vi "TagContainer-TestMain.vi"() -> ()   [LabVIEW 2017, in "TagDB(DEV).lvlib"]
uses:
  TagDB(DEV).lvlib
  a1ae43e1-b2e0-48b2-b5bf-09d8c6337ec0.vi
  5d4c14d8-f2b2-4cd0-9f9f-81160b0f88f4.vi
  69a5f5dc-289e-4520-a43d-4a6e53800127.vi
  f6a41f1a-46ba-40d5-b8b9-4f6d9d3cd2d0.vi
  b9594d6d-a8e1-4e69-b527-0d31d87043e6.vi
  _Support/DataAccess/_NameCacher.vi
  _Support/DataAccess/_datatypeChecker.vi
  _Support/DataAccess/TagDB Ref to DVR.vi
  <vilib>/Utility/Data Type/Get Type Information.vi
  <vilib>/Utility/error.llb/Trim Whitespace.vi
  _Support/Error/_[error50000]Invalid DB REF.vi
  _Support/Error/_[error50002]Invalid DataType.vi
  <userlib>/_OpenG.lib/comparison/comparison.llb/Variant Changed__ogtk.vi
  _Support/Change Detector/TagDB dbChanged.vi
panel:
  out "changed?":bool[](array[boolean])
  in  "Reject New Tag(F)":bool=TRUE
  out "should be datatype error":errorcluster
  out "should be no tag error":errorcluster
  out "Raw name":string
  in  "Type":cluster{"Numeric":i32, "String":string}
  in  "Stop":bool
  out "Value":cluster{"Numeric":i32, "String":string}
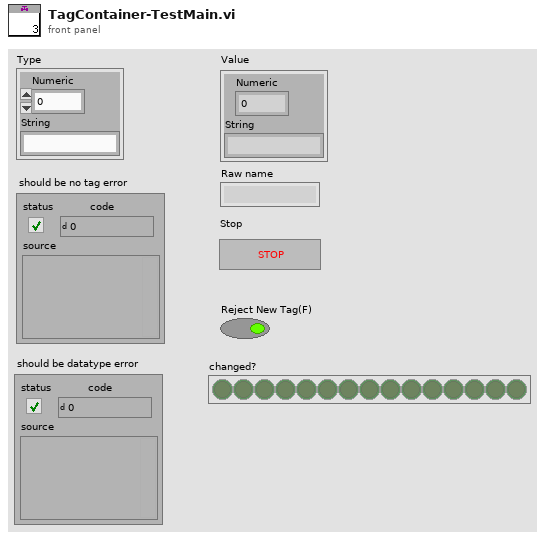
[diagram p1: front panel]
types:
  T1 = typedef "TagDB(DEV).lvlib/TagContainer.ctl" = refnum<k1>
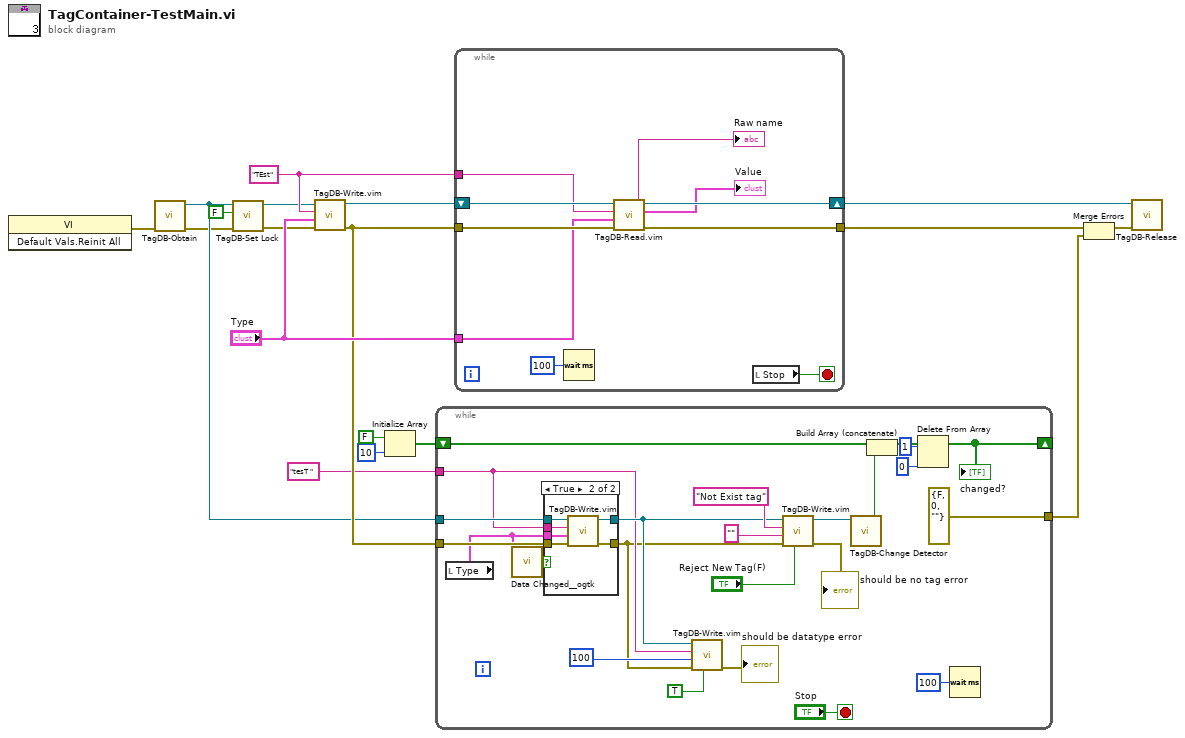
[diagram p0: block diagram]
diagram:
  w14 = "TEst" ("name")
  n1 = invoke class="VI" method="Default Vals.Reinit All"() -> (error out=w10:errorcluster)  [unwired: 3 in, 2 out]
  n2 = call "TagDB-Obtain.vi"("error in (no error)"=w10) -> ("error out"=w4:errorcluster, "TagContainer"=w5:T1)  [unwired: 4 in, 1 out]
  n3 = call "TagDB-Set Lock.vi"("error in (no error)"=w4, "Lock?(T)"=FALSE, "TagContainer"=w5) -> ("error out"=w3:errorcluster, "TagContainer(dup)"=w2:T1)  [unwired: 7 in]
  n4 = call "TagDB-Write.vim"("error in (no error)"=w3, "Value"="Type", "name"=w14, "TagContainer"=w2) -> ("error out"=w13:errorcluster, "TagContainer(dup)"=w18:T1)  [unwired: 5 in, 1 out]
  n5 = Initialize Array(FALSE, 10 ("dimension size")) -> (w6:bool[])
  n6 = while {
    tunnel: w5 -> [w40]
    tunnel: "tesT " ("name") -> [w33]
    tunnel: w13 -> [w39]
    tunnel: [errorcluster {"status"=FALSE, "code"=0, "source"=""} ("error out")] -> w11
    shift-right: [w24] -> _
    shift-left: w6 -> [w27]
    stop <- "Stop" stop-if-true
    n7 = local read "Type"() -> (w21:cluster{"Numeric":i32, "String":string})
    n8 = call-poly <userlib>:"Data Changed__ogtk.vi"("Variant"=w21) -> ("Changed"=w20:bool)
    n9 = case shown="True" w20 {
      tunnel: w40 -> [w44 w50]
      tunnel: w39 -> [w43 w49]
      tunnel: [w44 w48] -> w34
      tunnel: w33 -> [_ w47]
      tunnel: [w43 w46] -> w31
      tunnel: w21 -> [_ w45]
      frame False {
      }
      frame True {
        n10 = call "TagDB-Write.vim"("error in (no error)"=w49, "Value"=w45, "name"=w47, "TagContainer"=w50) -> ("error out"=w46:errorcluster, "TagContainer(dup)"=w48:T1)  [unwired: 5 in, 1 out]
      }
    }
    n11 = call "TagDB-Write.vim"("Reject New Tag(F)"=TRUE, "error in (no error)"=w31, "Value"=u32 100 ("milliseconds to wait"), "name"=w33, "TagContainer"=w34) -> ("error out"=→"should be datatype error":errorcluster)  [unwired: 4 in, 2 out]
    n12 = call "TagDB-Write.vim"("Reject New Tag(F)"="Reject New Tag(F)", "error in (no error)"=w31, "Value"="" ("name"), "name"="Not Exist tag", "TagContainer"=w34) -> ("error out"=→"should be no tag error":errorcluster, "TagContainer(dup)"=w28:T1)  [unwired: 4 in, 1 out]
    n13 = call-poly "TagDB-Change Detector.vi"("DB Ref"=w28) -> ("changed?"=w26:bool)  [unwired: 8 in, 2 out]
    n14 = Build Array (concatenate)(w27, w26) -> (w25:bool[])
    n15 = Delete From Array(array=w25, length=1, index=0) -> (array with subset deleted=w24:bool[])  [unwired: 1 out]
    "changed?" <- w24
    n16 = Wait (ms)(milliseconds to wait=u32 100) -> ()  [unwired: 1 out]
  }
  n17 = while {
    tunnel: w14 -> [w56]
    tunnel: "Type" -> [w55]
    shift-right: [w58] -> w17
    shift-left: w18 -> [w60]
    tunnel: w13 -> [w59]
    tunnel: [w57] -> w16
    stop <- w53 stop-if-true
    n18 = Wait (ms)(milliseconds to wait=u32 100) -> ()  [unwired: 1 out]
    n19 = call "TagDB-Read.vim"("error in (no error)"=w59, "Type"=w55, "name"=w56, "TagContainer"=w60) -> ("error out"=w57:errorcluster, "Value"=→"Value":cluster{"Numeric":i32, "String":string}, "TagContainer(dup)"=w58:T1, "Raw name"=→"Raw name":string)  [unwired: 2 in, 2 out]
    n20 = local read "Stop"() -> (w53:bool)
  }
  n21 = Merge Errors(w16, w11) -> (w12:errorcluster)
  n22 = call "TagDB-Release.vi"("error in (no error)"=w12, "TagContainer"=w17) -> ()  [unwired: 9 in, 1 out]
